vi "mousePositinToCursorPoistion.vi"(4 "Mouse Y position":i32, 5 "Mouse X position":i32, 7 "reference":refnum<vi>) -> (0 "Cursor Y position":dbl, 1 "Cursor X position":dbl, 2 "error out":errorcluster, 3 "reference out":refnum<vi>)   [LabVIEW 2014]
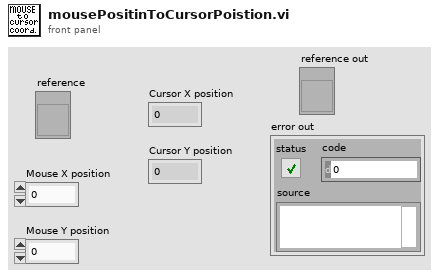
[diagram p1: front panel]
types:
  T1 = typedef "LVRangeTypeDef.ctl" = cluster{"Minimum":dbl, "Maximum":dbl, "Increment":dbl, "Minor Increment":dbl, "Start":dbl}
  T2 = typedef "LVRectTypeDef.ctl" = cluster{"Left":i16, "Top":i16, "Right":i16, "Bottom":i16}
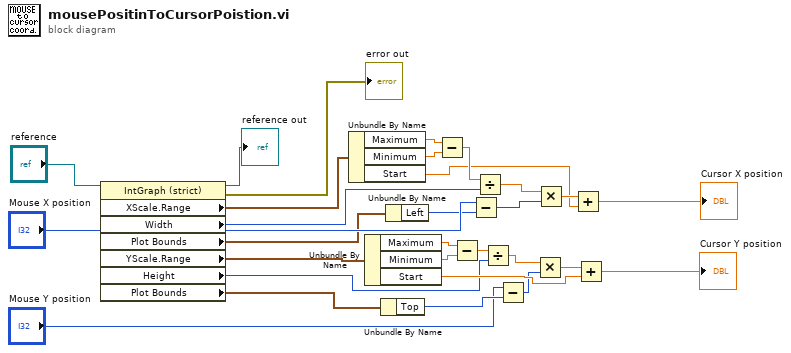
[diagram p0: block diagram]
diagram:
  n1 = property on="Property Node" class="IntGraph (strict)"(reference="reference") -> (reference out=→"reference out":refnum<vi>, error out=→"error out":errorcluster, "XScale.Range"=w16:T1, "Width"=w9:u32, "Plot Bounds"=w8:T2, "YScale.Range"=w19:T1, "Height"=w23:u32, "Plot Bounds"=w24:T2)  [unwired: 1 in]
  n2 = Unbundle By Name(w16) -> ("Maximum"=w15:dbl, "Minimum"=w14:dbl, "Start"=w6:dbl)
  n3 = Unbundle By Name(w19) -> ("Maximum"=w20:dbl, "Minimum"=w21:dbl, "Start"=w28:dbl)
  n4 = Unbundle By Name(w24) -> ("Top"=w2:i16)
  n5 = Unbundle By Name(w8) -> ("Left"=w7:i16)
  n6 = Subtract(x=w15, y=w14) -> (x-y=w13:dbl)
  n7 = Subtract(x=w20, y=w21) -> (x-y=w22:dbl)
  n8 = Subtract(x="Mouse X position", y=w7) -> (x-y=w11:i32)
  n9 = Divide(x=w13, y=w9) -> (x/y=w12:dbl)
  n10 = Divide(x=w22, y=w23) -> (x/y=w26:dbl)
  n11 = Subtract(x="Mouse Y position", y=w2) -> (x-y=w25:i32)
  n12 = Multiply(x=w26, y=w25) -> (x*y=w27:dbl)
  n13 = Multiply(x=w12, y=w11) -> (x*y=w10:dbl)
  n14 = Add(x=w10, y=w6) -> (x+y=→"Cursor X position":dbl)
  n15 = Add(x=w27, y=w28) -> (x+y=→"Cursor Y position":dbl)
